vi "niDTS WLAN UTIL Type to MCS Index.vi"(10 "WLAN Type":T1) -> (2 "MCS Index":i32)   [LabVIEW 2015, in "niDTS WLAN.lvlib"]
uses:
  niDTS WLAN.lvlib
  Includes/niDTS WLAN INC Type.ctl
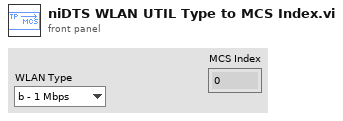
[diagram p1: front panel]
types:
  T1 = typedef "niDTS WLAN.lvlib/niDTS WLAN INC Type.ctl" = enum16{"b - 1 Mbps", "b - 2 Mbps", "b - 5.5 Mbps", "b - 11 Mbps", "ag - 6 Mbps", "ag - 9 Mbps", "ag - 12 Mbps", "ag - 18 Mbps", "ag - 24 Mbps", "ag - 36 Mbps", "ag - 48 Mbps", "ag - 54 Mbps", "n - MCS0", "n - MCS1", "n - MCS2", "n - MCS3", "n - MCS4", "n - MCS5", "n - MCS6", "n - MCS7", "n - MCS8", "n - MCS9", "n - MCS10", "n - MCS11", "n - MCS12", "n - MCS13", "n - MCS14", "n - MCS15", "n - MCS16", "n - MCS17", "n - MCS18", "n - MCS19", "n - MCS20", "n - MCS21", "n - MCS22", "n - MCS23", "n - MCS24", "n - MCS25", "n - MCS26", "n - MCS27", "n - MCS28", "n - MCS29", "n - MCS30", "n - MCS31", "ac - MCS0 -1", "ac - MCS1 -1", "ac - MCS2 -1", "ac - MCS3 -1", "ac - MCS4 -1", "ac - MCS5 -1", "ac - MCS6 -1", "ac - MCS7 -1", "ac - MCS8 -1", "ac - MCS9 -1", "ac - MCS0 -2", "ac - MCS1 -2", "ac - MCS2 -2", "ac - MCS3 -2", "ac - MCS4 -2", "ac - MCS5 -2", "ac - MCS6 -2", "ac - MCS7 -2", "ac - MCS8 -2", "ac - MCS9 -2", "ac - MCS0 -3", "ac - MCS1 -3", "ac - MCS2 -3", "ac - MCS3 -3", "ac - MCS4 -3", "ac - MCS5 -3", "ac - MCS6 -3", "ac - MCS7 -3", "ac - MCS8 -3", "ac - MCS9 -3", "ac - MCS0 -4", "ac - MCS1 -4", "ac - MCS2 -4", "ac - MCS3 -4", "ac - MCS4 -4", "ac - MCS5 -4", "ac - MCS6 -4", "ac - MCS7 -4", "ac - MCS8 -4", "ac - MCS9 -4"}
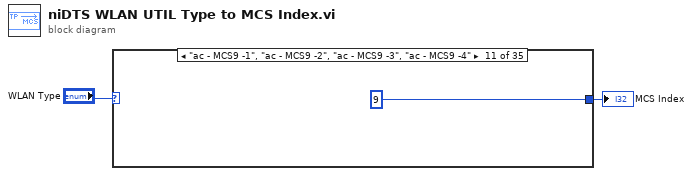
[diagram p0: block diagram]
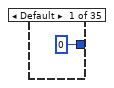
[diagram p2: hidden frame]
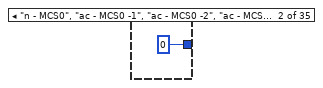
[diagram p3: hidden frame]
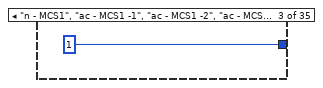
[diagram p4: hidden frame]
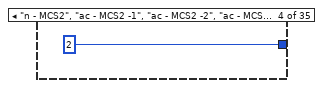
[diagram p5: hidden frame]
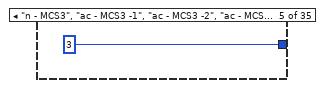
[diagram p6: hidden frame]
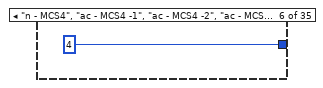
[diagram p7: hidden frame]
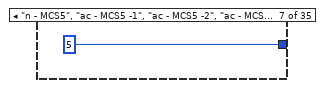
[diagram p8: hidden frame]
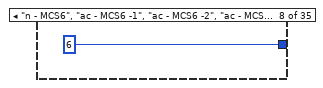
[diagram p9: hidden frame]
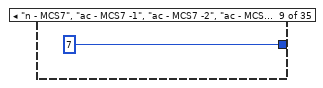
[diagram p10: hidden frame]
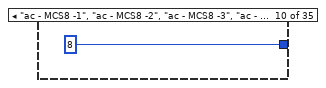
[diagram p11: hidden frame]
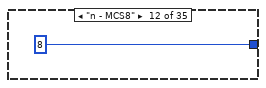
[diagram p12: hidden frame]
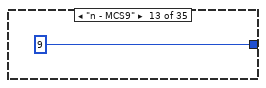
[diagram p13: hidden frame]
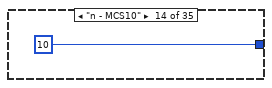
[diagram p14: hidden frame]
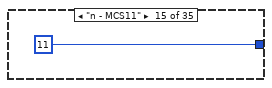
[diagram p15: hidden frame]
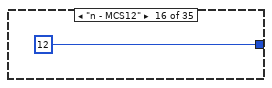
[diagram p16: hidden frame]
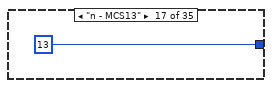
[diagram p17: hidden frame]
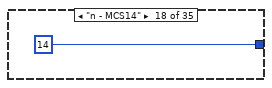
[diagram p18: hidden frame]
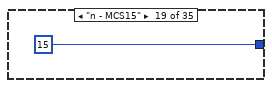
[diagram p19: hidden frame]
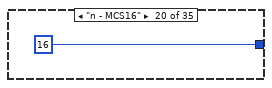
[diagram p20: hidden frame]
diagram:
  n1 = case shown="\"ac - MCS9 -1\", \"ac - MCS9 -2\", \"ac - MCS9 -3\", \"ac - MCS9 -4\"" "WLAN Type" {
    tunnel: [0 ("IQ.Header Detection") 0 ("IQ.Header Detection") 1 ("IQ.Header Detection") 2 ("IQ.Header Detection") 3 ("IQ.Header Detection") 4 ("IQ.Header Detection") 5 ("IQ.Header Detection") 6 ("IQ.Header Detection") 7 ("IQ.Header Detection") 8 ("IQ.Header Detection") 9 ("IQ.Header Detection") 8 ("IQ.Header Detection") 9 ("IQ.Header Detection") 10 ("IQ.Header Detection") 11 ("IQ.Header Detection") 12 ("IQ.Header Detection") 13 ("IQ.Header Detection") 14 ("IQ.Header Detection") 15 ("IQ.Header Detection") 16 ("IQ.Header Detection") 17 ("IQ.Header Detection") 18 ("IQ.Header Detection") 19 ("IQ.Header Detection") 20 ("IQ.Header Detection") 21 ("IQ.Header Detection") 22 ("IQ.Header Detection") 23 ("IQ.Header Detection") 24 ("IQ.Header Detection") 25 ("IQ.Header Detection") 26 ("IQ.Header Detection") 27 ("IQ.Header Detection") 28 ("IQ.Header Detection") 29 ("IQ.Header Detection") 30 ("IQ.Header Detection") 31 ("IQ.Header Detection")] -> w1
    frame Default {
    }
    frame "n - MCS0", "ac - MCS0 -1", "ac - MCS0 -2", "ac - MCS0 -3", "ac - MCS0 -4" {
    }
    frame "n - MCS1", "ac - MCS1 -1", "ac - MCS1 -2", "ac - MCS1 -3", "ac - MCS1 -4" {
    }
    frame "n - MCS2", "ac - MCS2 -1", "ac - MCS2 -2", "ac - MCS2 -3", "ac - MCS2 -4" {
    }
    frame "n - MCS3", "ac - MCS3 -1", "ac - MCS3 -2", "ac - MCS3 -3", "ac - MCS3 -4" {
    }
    frame "n - MCS4", "ac - MCS4 -1", "ac - MCS4 -2", "ac - MCS4 -3", "ac - MCS4 -4" {
    }
    frame "n - MCS5", "ac - MCS5 -1", "ac - MCS5 -2", "ac - MCS5 -3", "ac - MCS5 -4" {
    }
    frame "n - MCS6", "ac - MCS6 -1", "ac - MCS6 -2", "ac - MCS6 -3", "ac - MCS6 -4" {
    }
    frame "n - MCS7", "ac - MCS7 -1", "ac - MCS7 -2", "ac - MCS7 -3", "ac - MCS7 -4" {
    }
    frame "ac - MCS8 -1", "ac - MCS8 -2", "ac - MCS8 -3", "ac - MCS8 -4" {
    }
    frame "ac - MCS9 -1", "ac - MCS9 -2", "ac - MCS9 -3", "ac - MCS9 -4" {
    }
    frame "n - MCS8" {
    }
    frame "n - MCS9" {
    }
    frame "n - MCS10" {
    }
    frame "n - MCS11" {
    }
    frame "n - MCS12" {
    }
    frame "n - MCS13" {
    }
    frame "n - MCS14" {
    }
    frame "n - MCS15" {
    }
    frame "n - MCS16" {
    }
    frame "n - MCS17" {
    }
    frame "n - MCS18" {
    }
    frame "n - MCS19" {
    }
    frame "n - MCS20" {
    }
    frame "n - MCS21" {
    }
    frame "n - MCS22" {
    }
    frame "n - MCS23" {
    }
    frame "n - MCS24" {
    }
    frame "n - MCS25" {
    }
    frame "n - MCS26" {
    }
    frame "n - MCS27" {
    }
    frame "n - MCS28" {
    }
    frame "n - MCS29" {
    }
    frame "n - MCS30" {
    }
    frame "n - MCS31" {
    }
  }
  "MCS Index" <- w1
